vi "delta_j.vi"(0 "w_jk_2":dbl, 1 "w_jk_1":dbl, 5 "w_jk_3":dbl, 7 "O_j":dbl, 9 "delta_k_1":dbl, 11 "delta_k_2":dbl, 12 "delta_k_3":dbl) -> (8 "delta_j":dbl)   [LabVIEW 2014]
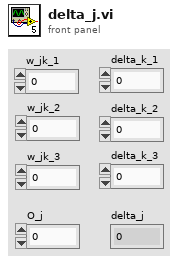
[diagram p1: front panel]
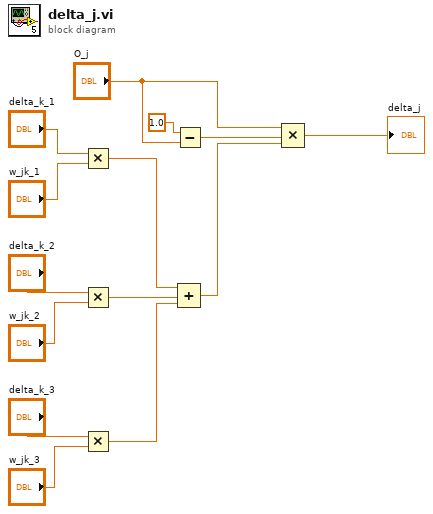
[diagram p0: block diagram]
diagram:
  n1 = Multiply(x="delta_k_1", y="w_jk_1") -> (x*y=w4:dbl)
  n2 = Multiply(x="delta_k_2", y="w_jk_2") -> (x*y=w3:dbl)
  n3 = Multiply(x="delta_k_3", y="w_jk_3") -> (x*y=w2:dbl)
  n4 = Subtract(x=1.0, y="O_j") -> (x-y=w12:dbl)
  n5 = Compound Arithmetic op=ADD(w4, w3, w2) -> (w1:dbl)
  n6 = Compound Arithmetic op=MULTIPLY("O_j", w12, w1) -> (→"delta_j":dbl)
